vi "RSLIP gait.vi"(0 "gait Data":T1, 1 "Buffer Ratio":dbl, 2 "Input Time":dbl) -> (11 "t (mode)":dbl, 15 "Set Point":dbl, 16 "Set Point (V)":dbl, 17 "state":dbl)   [LabVIEW 2019]
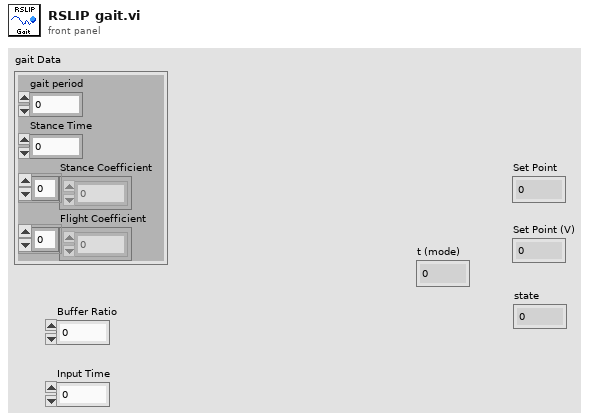
[diagram p1: front panel]
types:
  T1 = cluster{"gait period":dbl, "Stance Time":dbl, "Stance Coefficient":dbl[], "Flight Coefficient":dbl[]}
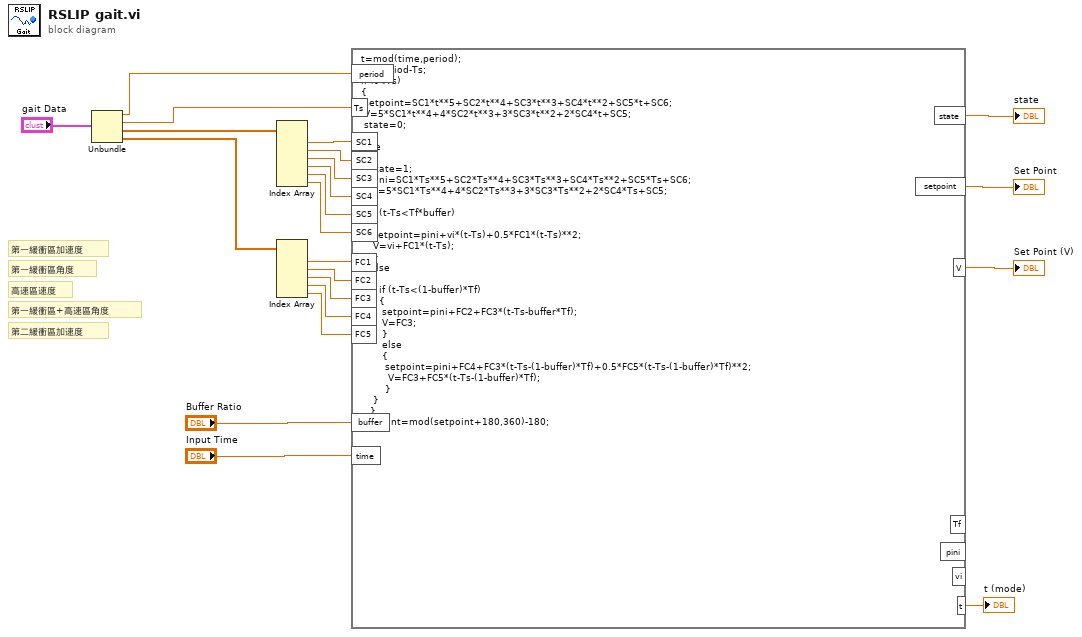
[diagram p0: block diagram]
diagram:
  # "第二緩衝區加速度"
  # "第一緩衝區+高速區角度"
  # "高速區速度"
  # "第一緩衝區角度"
  # "第一緩衝區加速度"
  n1 = Unbundle("gait Data") -> ("gait period"=w7:dbl, "Stance Time"=w6:dbl, "Stance Coefficient"=w5:dbl[], "Flight Coefficient"=w4:dbl[])
  n2 = Index Array(array=w5) -> (element #1=w22:dbl, element #2=w21:dbl, element #3=w20:dbl, element #4=w19:dbl, element #5=w18:dbl, element #6=w17:dbl)  [unwired: 6 in]
  n3 = Index Array(array=w4) -> (element #1=w16:dbl, element #2=w15:dbl, element #3=w14:dbl, element #4=w13:dbl, element #5=w12:dbl)  [unwired: 5 in]
  n4 = formula code="t=mod(time,period);\nTf=period-Ts;\nif (t<Ts)\n{\n setpoint=SC1*t**5+SC2*t**4+SC3*t**3+SC4*t**2+SC5*t+SC6;\n V=5*SC1*t**4+4*SC2*t**3+3*SC3*t**2+2*SC4*t+SC5;\n state=0;\n}\nelse\n{\n   state=1;\n   pini=SC1*Ts**5+SC2*Ts**4+SC3*Ts**3+SC4*Ts**2+SC5*Ts+SC6;\n   vi=5*SC1*Ts**4+4*SC2*Ts**3+3*SC3*Ts**2+2*SC4*Ts+SC5;\n  \n   if (t-Ts<Tf*buffer)\n  {\n    setpoint=pini+vi*(t-Ts)+0.5*FC1*(t-Ts)**2;\n    V=vi+FC1*(t-Ts);\n    }\n   else\n   {\n      if (t-Ts<(1-buffer)*Tf) \n      {\n       setpoint=pini+FC2+FC3*(t-Ts-buffer*Tf);\n       V=FC3;\n       }\n       else\n       {\n        setpoint=pini+FC4+FC3*(t-Ts-(1-buffer)*Tf)+0.5*FC5*(t-Ts-(1-buffer)*Tf)**2;\n         V=FC3+FC5*(t-Ts-(1-buffer)*Tf);\n        }\n    } \n   }\nsetpoint=mod(setpoint+180,360)-180;"("period"=w7, "Ts"=w6, "SC1"=w22, "SC2"=w21, "SC3"=w20, "SC4"=w19, "SC5"=w18, "SC6"=w17, "FC1"=w16, "FC2"=w15, "FC3"=w14, "FC4"=w13, "FC5"=w12, "buffer"="Buffer Ratio", "time"="Input Time") -> ("setpoint"=→"Set Point":dbl, "t"=→"t (mode)":dbl, "V"=→"Set Point (V)":dbl, "state"=→"state":dbl)  [unwired: 3 out]
